vi "Finish.vi"(6 "Sender":refnum<class "Sender.lvclass">, 9 "Error":errorcluster, 10 "Actor":refnum<class "Actor.lvclass">, 11 "TEMPLATE Actor in":refnum<class "TEMPLATE Actor.lvclass">) -> (0 "Error out":errorcluster, 3 "TEMPLATE Actor out":refnum<class "TEMPLATE Actor.lvclass">)   [LabVIEW 2025, in "_Template.lvlib" / "Templates.lvlib" / "TEMPLATE Actor.lvlib" / "TEMPLATE Actor.lvclass"]
uses:
  TEMPLATE Actor.lvclass
  jettl/jettl/Actor/Actor/Actor.lvclass
  jettl/jettl/Sender/Sender/Sender.lvclass
  TEMPLATE Actor.lvclass/TEMPLATE Actor.ctl
  jettl/jettl/Finish Msg/Decorator.vi
  jettl/jettl/Finish Msg/Finish Msg.lvlib
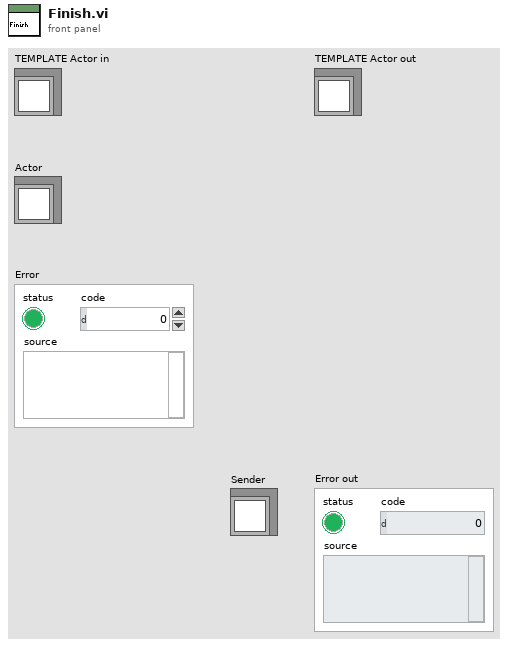
[diagram p1: front panel]
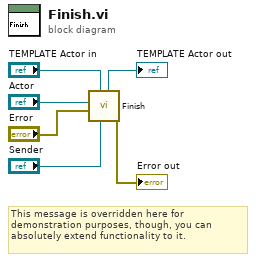
[diagram p0: block diagram]
diagram:
  # "This message is overridden here for demonstration purposes, though, you can absolutely extend functionality to it."
  n1 = call-poly "Finish.vi"("Sender"="Sender", "Actor in"="TEMPLATE Actor in", "Error"="Error", "Actor"="Actor") -> ("Error out"=→"Error out":errorcluster, "Actor out"=→"TEMPLATE Actor out":refnum<class "TEMPLATE Actor.lvclass">)  [unwired: 6 in]
